vi "Read Default From File.vi"(8 "error in (no error)":errorcluster, 9 "Name":string, 10 "Path":path, 11 "Funnel Settings in":refnum<class "Funnel Settings.lvclass">) -> (0 "error out":errorcluster, 3 "Funnel Settings out":refnum<class "Funnel Settings.lvclass">)   [LabVIEW 2019, in "Funnel Settings.lvclass"]
uses:
  Funnel Settings.lvclass
  ObjectSettings/ObjectSettings.lvclass
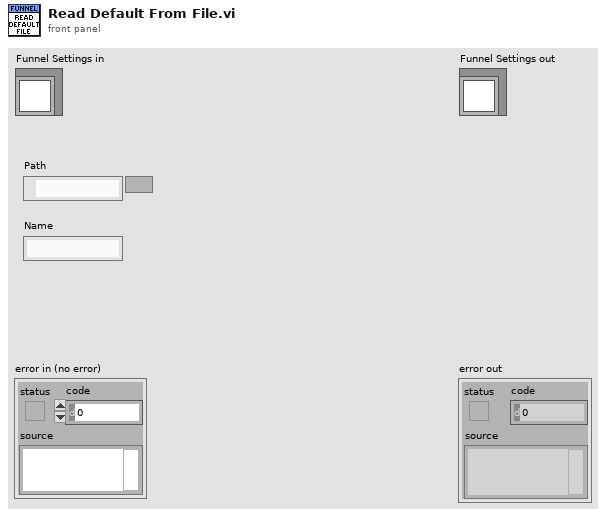
[diagram p1: front panel]
types:
  T1 = typedef "Funnel Settings.lvclass/Default Funnel Cluster.ctl" = cluster{"Smooth Segments":dbl, "Bottom Segments":dbl}
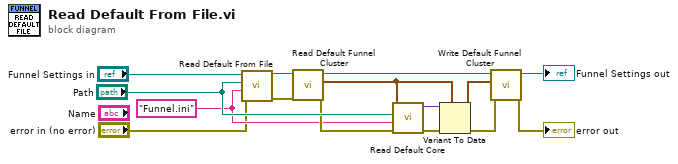
[diagram p0: block diagram]
diagram:
  w2 = "Funnel.ini"
  n1 = call-parent "Read Default From File.vi"("error in (no error)"="error in (no error)", "Name"=w2, "Path"="Path", "ObjectSettings in"="Funnel Settings in") -> ("error out"=w7:errorcluster, "ObjectSettings out"=w13:refnum<class "Funnel Settings.lvclass">)  [unwired: 6 in]
  n2 = call "Read Default Funnel Cluster.vi"("error in (no error)"=w7, "Funnel Settings in"=w13) -> ("error out"=w9:errorcluster, "Default Funnel"=w5:T1, "Funnel Settings out"=w14:refnum<class "Funnel Settings.lvclass">)  [unwired: 7 in]
  n3 = call "Read Default Core.vi"("error in (no error)"=w9, "Name"=w2, "Path"="Path", "Cluster In"=w5) -> ("error out"=w8:errorcluster, "Cluster Out"=w10:variant)  [unwired: 6 in]
  n4 = Variant To Data(error in=w8, type=w5, Variant=w10) -> (data=w6:T1, error out=w4:errorcluster)
  n5 = call "Write Default Funnel Cluster.vi"("error in (no error)"=w4, "Default Funnel"=w6, "Funnel Settings in"=w14) -> ("error out"=→"error out":errorcluster, "Funnel Settings out"=→"Funnel Settings out":refnum<class "Funnel Settings.lvclass">)  [unwired: 7 in]
